vi "Create_Object.vi"(8 "error in (no error)":errorcluster, 9 "Terminal Map in":map{string, T1}(c390), 10 "owner refnum":variant, 11 "Numeric Control in":refnum<class "Numeric Control.lvclass">) -> (0 "error out":errorcluster, 1 "Terminal Map Out":map{string, T1}(c390), 3 "Numeric Control out":refnum<class "Numeric Control.lvclass">)   [LabVIEW 2025, in "Numeric Control.lvclass"]
uses:
  Numeric Control.lvclass
  C:/Users/mrjak/Documents/GitHub/LVGPT/LabVIEW/VIs/Classes/Node/Node.lvclass
  Terminal.ctl
  <vilib>/numeric/LVNumericRepresentation.ctl
  Node.lvclass/Node.ctl
  Control.lvclass
  Numeric Control.lvclass/Numeric Control.ctl
  Node.lvclass
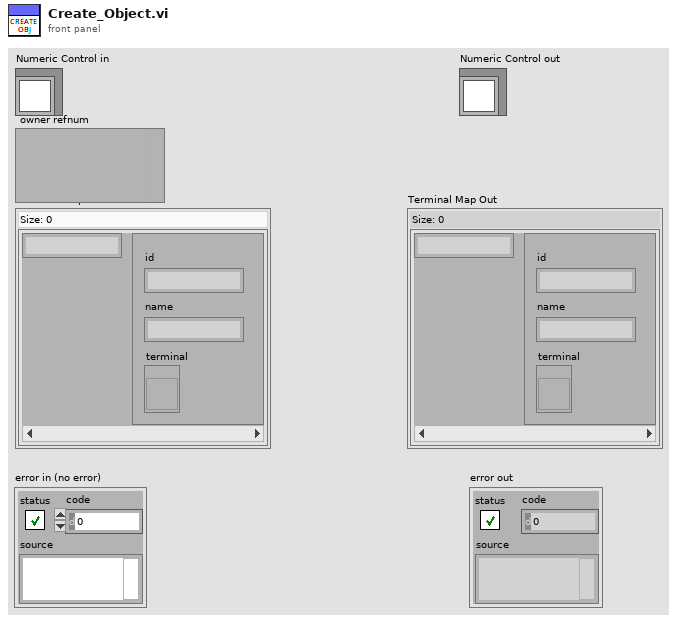
[diagram p1: front panel]
types:
  T1 = typedef "Terminal.ctl" = cluster{"id":string, "name":string, "terminal":refnum<vi>}
  T2 = typedef "LVNumericRepresentation.ctl" = enum32{"Extended Precision", "Double Precision", "Single Precision", "Long", "Word", "Byte", "Unsigned Long", "Unsigned Word", "Unsigned Byte", "Complex Extended", "Complex Double", "Complex Single", "Quad", "Unsigned Quad", "Fixed-Point"}
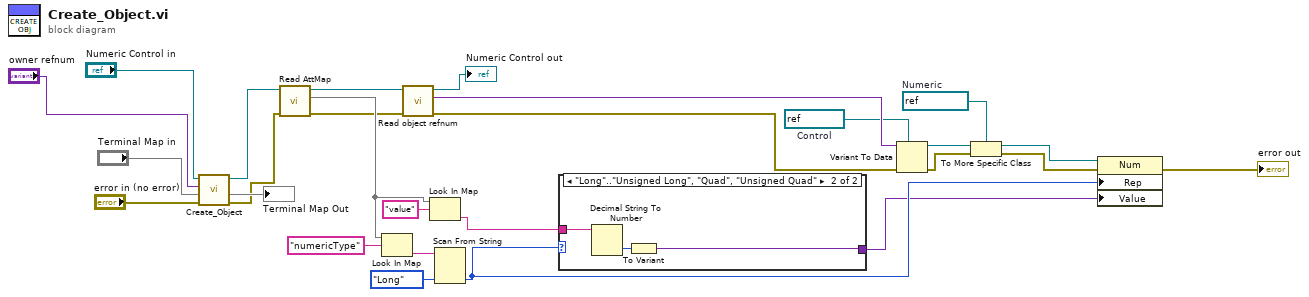
[diagram p0: block diagram]
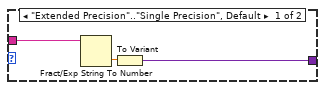
[diagram p2: hidden frame]
diagram:
  w10 = refnum<vi> refnum  # Numeric
  w14 = refnum<vi> refnum  # Control
  n1 = call-parent "Create_Object.vi"("error in (no error)"="error in (no error)", "Terminal Map in"="Terminal Map in", "owner refnum"="owner refnum", "Control in"="Numeric Control in") -> ("error out"=w4:errorcluster, "Terminal Map Out"=→"Terminal Map Out":map{string, T1}, "Control out"=w5:refnum<class "Numeric Control.lvclass">)  [unwired: 5 in]
  n2 = call "Read AttMap.vi"("error in (no error)"=w4, "Node in"=w5) -> ("error out"=w16:errorcluster, "AttMap"=w19:map{string, string}, "Node out"=w17:refnum<class "Numeric Control.lvclass">)  [unwired: 7 in]
  n3 = Look In Map(map=w19, key="numericType") -> (value=w21:string)  [unwired: 1 in, 1 out]
  n4 = call-dynamic "Read object refnum.vi"("error in (no error)"=w16, "Node in"=w17) -> ("error out"=w12:errorcluster, "object refnum"=w15:variant, "Node out"=→"Numeric Control out":refnum<class "Numeric Control.lvclass">)  [unwired: 7 in]
  n5 = Look In Map(map=w19, key="value") -> (value=w18:string)  [unwired: 1 in, 1 out]
  n6 = Scan From String(input string=w21, default 1=LVNumericRepresentation."Long" ("Representation")) -> (output 1=w7:T2)  [unwired: 3 in, 3 out]
  n7 = case shown="\"Long\"..\"Unsigned Long\", \"Quad\", \"Unsigned Quad\"" w7 {
    tunnel: w18 -> [w30 w33]
    tunnel: [w28 w31] -> w6
    frame "Extended Precision".."Single Precision", Default {
      n8 = Fract/Exp String To Number(string=w30) -> (number=w29:dbl)  [unwired: 3 in, 1 out]
      n9 = To Variant(anything=w29) -> (Variant=w28:variant)
    }
    frame "Long".."Unsigned Long", "Quad", "Unsigned Quad" {
      n10 = Decimal String To Number(string=w33) -> (number=w32:i32)  [unwired: 2 in, 1 out]
      n11 = To Variant(anything=w32) -> (Variant=w31:variant)
    }
  }
  n12 = Variant To Data(error in=w12, type=w14, Variant=w15) -> (data=w13:refnum<vi>, error out=w9:errorcluster)
  n13 = To More Specific Class(target class=w10, reference=w13, error in=w9) -> (specific class reference=w11:refnum<vi>, error out=w8:errorcluster)
  n14 = property class="Num"(reference=w11, error in=w8, "Rep"=w7, "Value"=w6) -> (error out=→"error out":errorcluster)  [unwired: 1 out]
